vi "Actor Core.vi"(8 "error in":errorcluster, 11 "Pulse Configuration in":refnum<class "Pulse Configuration.lvclass">) -> (0 "error out":errorcluster, 3 "Actor out":refnum<class "Actor.lvclass">)   [LabVIEW 2015, in "Pulse Configuration.lvclass"]
doc: "(<B>Filename</B>: Actor Framework.lvlib:Actor.lvclass:Actor Core.vi)\n\nReceives messages to the actor, reacts to them, and initiates any error handling that may shut the actor down.\n\nDescendant classes may override this VI to append parallel tasks for the actor to complete while it handles messages. Overrides use the Call Parent Method node."
uses:
  Pulse Configuration.lvclass
  <vilib>/ActorFramework/Actor/Actor.lvclass
  Measure Object/Measure Object.lvclass
panel:
  in  "Configuration":T1={"Pre-trigger duration"=-1.0, "Post-trigger duration"=-1.0} {"Pre-trigger duration" format="%#_6p"; "Post-trigger duration" format="%#_6p"}
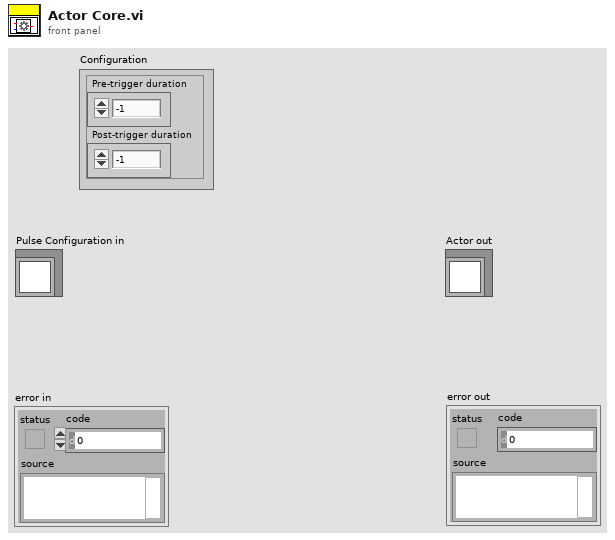
[diagram p1: front panel]
types:
  T1 = cluster{"Pre-trigger duration":dbl, "Post-trigger duration":dbl}
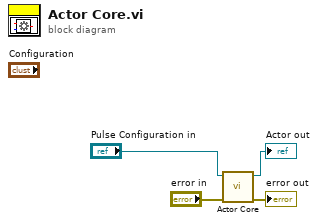
[diagram p0: block diagram]
diagram:
  n1 = call-parent "Actor Core.vi"("error in"="error in", "Measure Object in"="Pulse Configuration in") -> ("error out"=→"error out":errorcluster, "Actor out"=→"Actor out":refnum<class "Actor.lvclass">)  [unwired: 8 in]
